vi "Host_Main.vi"() -> ()   [LabVIEW 2017]
doc: "Vi pozwala na podstawowe komunikowanie się użytkownika z urządzeniem, przesyłanie danych pomiędzy RT, a Hostem oraz obserwowanie ostatecznego wyniku kąta padania dźwięku na urządzenie."
uses:
  Custom Controls/#typedef_Angle Indicator.ctl
panel:
  out "Error Out":errorcluster
  out "Signal":dbl[](graph)
  out "TDOA":dbl[](graph)
  out "SingleAngleError?":bool
  out "FatalAngleError?":bool
  in  "Threshold":fxp<+/-,28,9>=0.10000038146972656
  in  "SamplesToSend":u32=9000
  in  "AcqLoopFreq(kS/s)":dbl=50.0
  out "FIFO Timeout?":bool
  out "Angle_Gauge":T1 scale=-90.0..90.0
  in  "Stop":bool
  # "Errors"
  # "Signals"
  # "Settings"
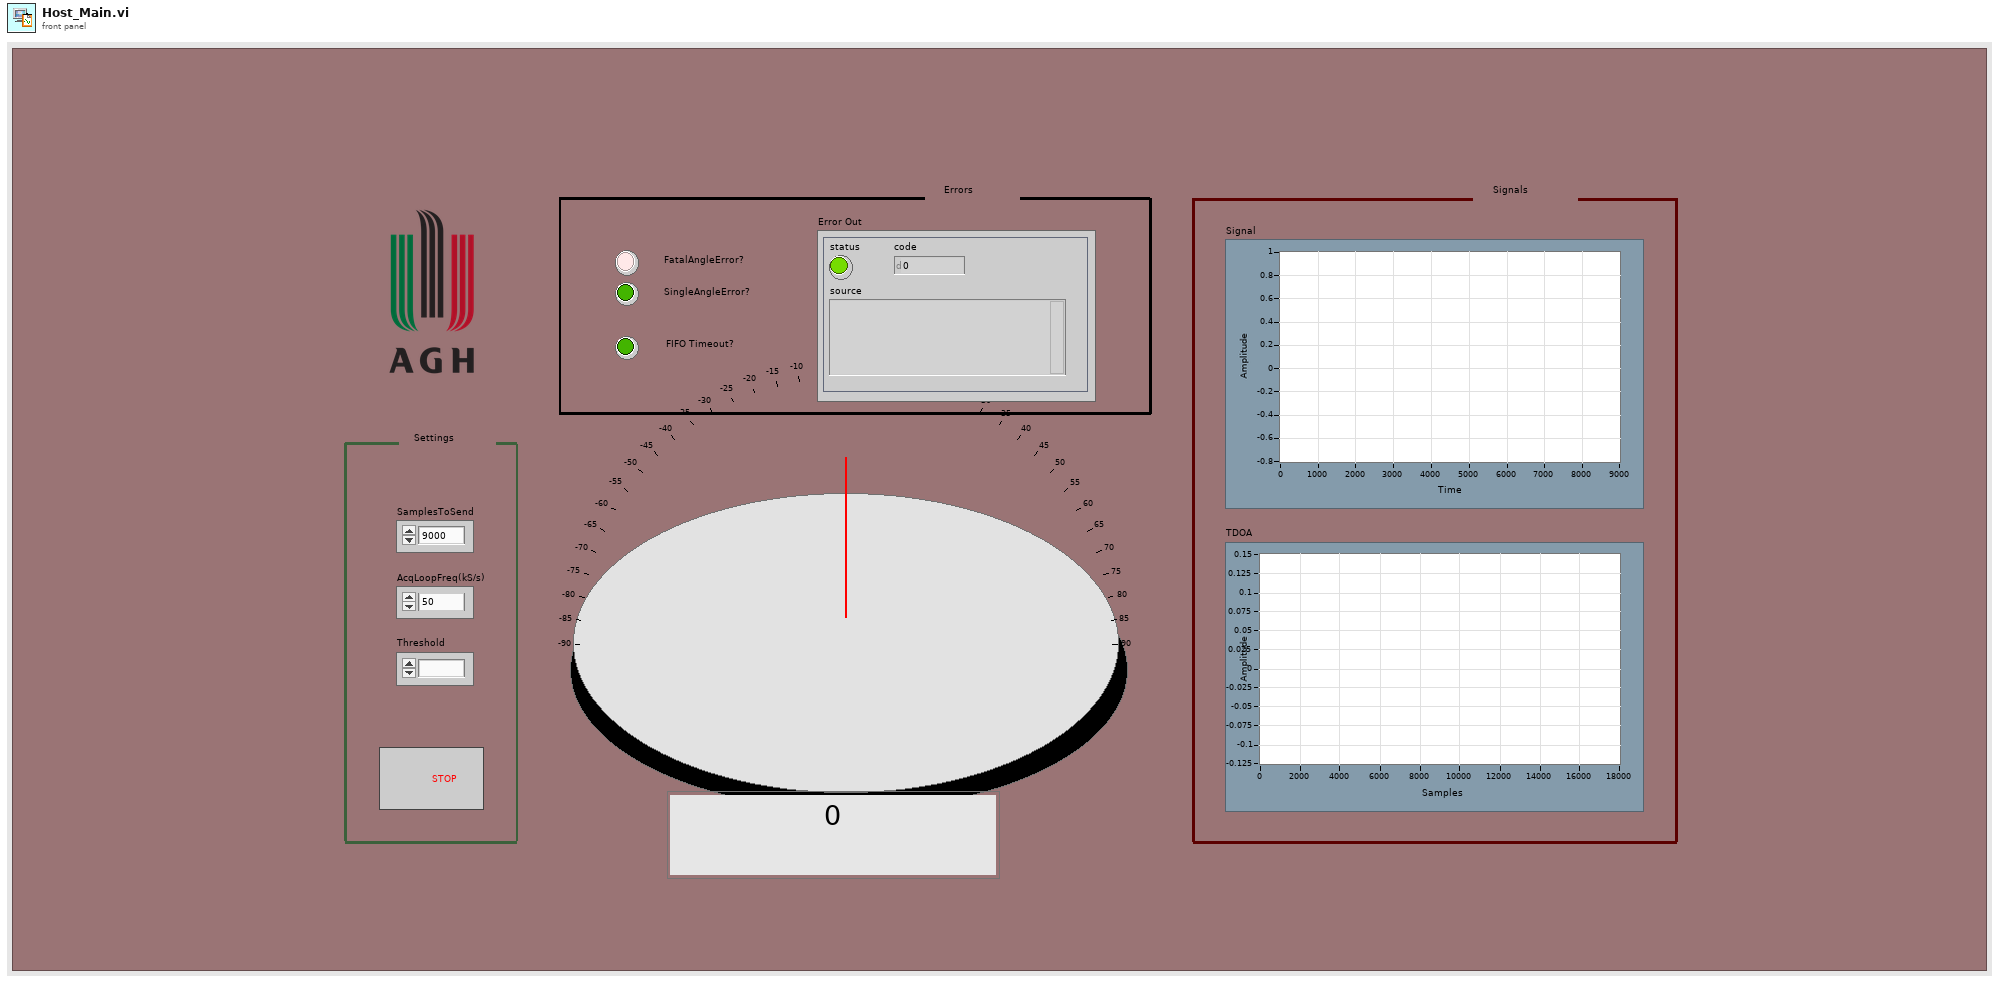
[diagram p1: front panel]
types:
  T1 = typedef "#typedef_Angle Indicator.ctl" = dbl
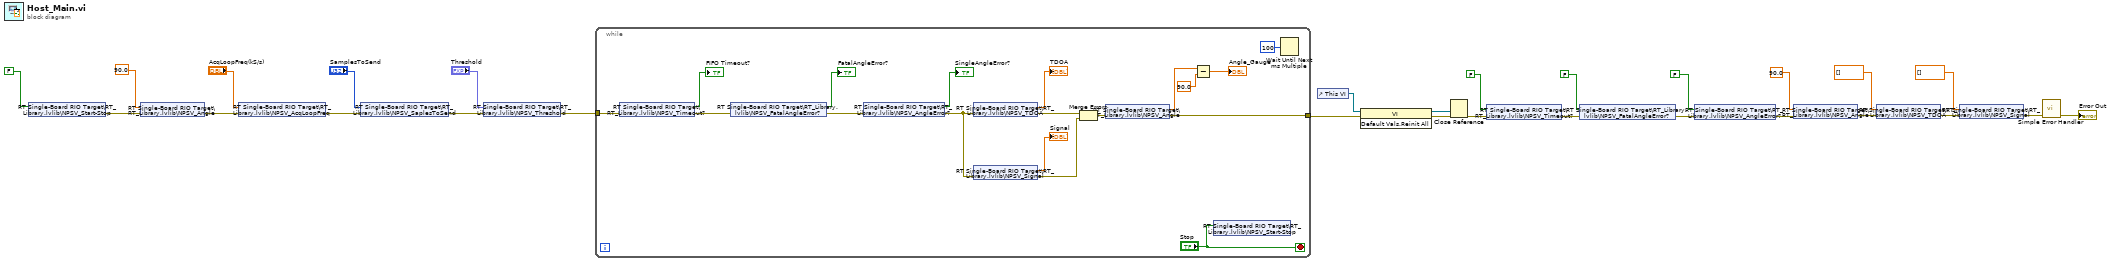
[diagram p0: block diagram]
diagram:
  n1 = shared-variable "RT Single-Board RIO Target\\RT_Library.lvlib\\NPSV_Start-Stop"(FALSE ("NPSV_Start-Stop")) -> (error out=w2:errorcluster)  [unwired: 1 in]
  n2 = shared-variable "RT Single-Board RIO Target\\RT_Library.lvlib\\NPSV_Angle"(90.0 ("NPSV_Angle"), error in=w2) -> (error out=w1:errorcluster)
  n3 = shared-variable "RT Single-Board RIO Target\\RT_Library.lvlib\\NPSV_AcqLoopFreq"("AcqLoopFreq(kS/s)", error in=w1) -> (error out=w21:errorcluster)
  n4 = shared-variable "RT Single-Board RIO Target\\RT_Library.lvlib\\NPSV_SaplesToSend"("SamplesToSend", error in=w21) -> (error out=w20:errorcluster)
  n5 = shared-variable "RT Single-Board RIO Target\\RT_Library.lvlib\\NPSV_Threshold"("Threshold", error in=w20) -> (error out=w19:errorcluster)
  n6 = while {
    tunnel: w19 -> [w38]
    tunnel: [w29] -> w4
    stop <- "Stop" stop-if-true
    n7 = shared-variable "RT Single-Board RIO Target\\RT_Library.lvlib\\NPSV_Timeout?"(error in=w38) -> (→"FIFO Timeout?":bool, error out=w37:errorcluster)
    n8 = shared-variable "RT Single-Board RIO Target\\RT_Library.lvlib\\NPSV_FatalAngleError?"(error in=w37) -> (→"FatalAngleError?":bool, error out=w36:errorcluster)
    n9 = shared-variable "RT Single-Board RIO Target\\RT_Library.lvlib\\NPSV_AngleError?"(error in=w36) -> (→"SingleAngleError?":bool, error out=w34:errorcluster)
    n10 = shared-variable "RT Single-Board RIO Target\\RT_Library.lvlib\\NPSV_TDOA"(error in=w34) -> (→"TDOA":dbl[], error out=w31:errorcluster)
    n11 = shared-variable "RT Single-Board RIO Target\\RT_Library.lvlib\\NPSV_Signal"(error in=w34) -> (→"Signal":dbl[], error out=w30:errorcluster)
    n12 = Merge Errors(w31, w30) -> (w32:errorcluster)
    n13 = shared-variable "RT Single-Board RIO Target\\RT_Library.lvlib\\NPSV_Angle"(error in=w32) -> (w45:dbl, error out=w29:errorcluster)
    n14 = Subtract(x=w45, y=90.0) -> (x-y=→"Angle_Gauge":dbl)
    n15 = shared-variable "RT Single-Board RIO Target\\RT_Library.lvlib\\NPSV_Start-Stop"("Stop") -> ()  [unwired: 1 in, 1 out]
    n16 = Wait Until Next ms Multiple(millisecond multiple=u32 100) -> ()  [unwired: 1 out]
  }
  n17 = control-ref of="This VI"() -> (w8:refnum<vi>)
  n18 = invoke class="VI" method="Default Vals.Reinit All"(reference=w8, error in=w4) -> (reference out=w6:refnum<vi>, error out=w7:errorcluster)  [unwired: 1 in, 1 out]
  n19 = Close Reference(reference=w6, error in (no error)=w7) -> (error out=w5:errorcluster)
  n20 = shared-variable "RT Single-Board RIO Target\\RT_Library.lvlib\\NPSV_Timeout?"(FALSE ("NPSV_Timeout?"), error in=w5) -> (error out=w11:errorcluster)
  n21 = shared-variable "RT Single-Board RIO Target\\RT_Library.lvlib\\NPSV_FatalAngleError?"(FALSE ("NPSV_NaN?"), error in=w11) -> (error out=w10:errorcluster)
  n22 = shared-variable "RT Single-Board RIO Target\\RT_Library.lvlib\\NPSV_AngleError?"(FALSE ("NPSV_NaN?"), error in=w10) -> (error out=w9:errorcluster)
  n23 = shared-variable "RT Single-Board RIO Target\\RT_Library.lvlib\\NPSV_Angle"(90.0 ("NPSV_Angle"), error in=w9) -> (error out=w15:errorcluster)
  n24 = shared-variable "RT Single-Board RIO Target\\RT_Library.lvlib\\NPSV_TDOA"(dbl[] [] ("NPSV_TDOA"), error in=w15) -> (error out=w13:errorcluster)
  n25 = shared-variable "RT Single-Board RIO Target\\RT_Library.lvlib\\NPSV_Signal"(dbl[] [] ("NPSV_Signal"), error in=w13) -> (error out=w14:errorcluster)
  n26 = call <vilib>:"Simple Error Handler.vi"("error in (no error)"=w14) -> ("error out"=→"Error Out":errorcluster)  [unwired: 4 in, 4 out]
